vi "iWorx Polar Pulse SubVI.vi"(7 "Waveform Chart Ref":refnum<vi>, 10 "Threashold":dbl) -> (0 "Pulse Times":timestamp[](array[timestamp]), 1 "Inst Pulse Rate":dbl, 2 "Avg Pulse Rate":dbl)   [LabVIEW 2014]
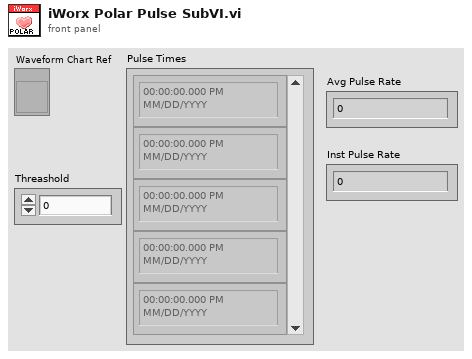
[diagram p1: front panel]
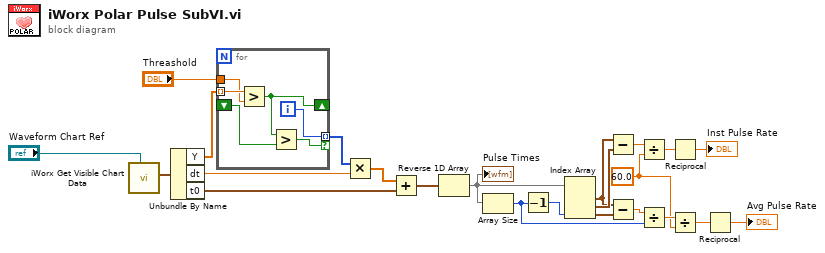
[diagram p0: block diagram]
diagram:
  w5 = 60.0 ("y")
  n1 = call "iWorx Get Visible Chart Data.vi"("Selection Chart"="Waveform Chart Ref") -> ("Waveform out"=w23:waveform(dbl))  [unwired: 8 in, 2 out]
  n2 = Unbundle By Name(w23) -> ("Y"=w21:dbl[], "dt"=w18:dbl, "t0"=w20:timestamp)
  n3 = for {
    tunnel: w21 -> [w29] mode=indexing
    tunnel: [w28] -> w17 mode=indexing if=w24
    tunnel: "Threashold" -> [w27]
    shift-right: [w26] -> _
    shift-left: _ -> [w25]
    i -> [w28]
    n4 = Greater?(x=w29, y=w27) -> (0:w26:bool)
    n5 = Greater?(x=w26, y=w25) -> (0:w24:bool)
  }
  n6 = Multiply(x=w17, y=w18) -> (x*y=w19:dbl[])
  n7 = Add(x=w19, y=w20) -> (x+y=w15:timestamp[])
  n8 = Reverse 1D Array(array=w15) -> (reversed array=w13:timestamp[])
  "Pulse Times" <- w13
  n9 = Array Size(array=w13) -> (size(s)=w8:i32)
  n10 = Decrement(x=w8) -> (x-1=w12:i32)
  n11 = Index Array(array=w13, index #3=w12) -> (element #1=w11:timestamp, element #2=w14:timestamp, element #3=w10:timestamp)  [unwired: 2 in]
  n12 = Subtract(x=w11, y=w14) -> (x-y=w6:dbl)
  n13 = Subtract(x=w11, y=w10) -> (x-y=w9:dbl)
  n14 = Divide(x=w6, y=w5) -> (x/y=w4:dbl)
  n15 = Divide(x=w9, y=w8) -> (x/y=w7:dbl)
  n16 = Reciprocal(x=w4) -> (1/x=→"Inst Pulse Rate":dbl)
  n17 = Divide(x=w7, y=w5) -> (x/y=w3:dbl)
  n18 = Reciprocal(x=w3) -> (1/x=→"Avg Pulse Rate":dbl)
